vi "Data Producer Worker Template_Read.vi"(0 "Data Producer Worker Template In":refnum<class "Data Producer Worker Template.lvclass">, 7 "Elements to Read (-1: all)":i32=-1) -> (4 "Data Producer Worker Template Out":refnum<class "Data Producer Worker Template.lvclass">)   [LabVIEW 2013, in "Data Producer Worker Template.lvclass"]
uses:
  Data Producer Worker Template.lvclass
  Data Producer Worker Template.lvclass/Data Producer Worker Template.ctl
panel:
  out "Timeout":bool
  out "Elements Remaining":i32
  out "error out":errorcluster
  in  "error in (no error)":errorcluster
  in  "timeout in ms (-1)":i32=-1
  out "Data":dbl[](array[numeric])
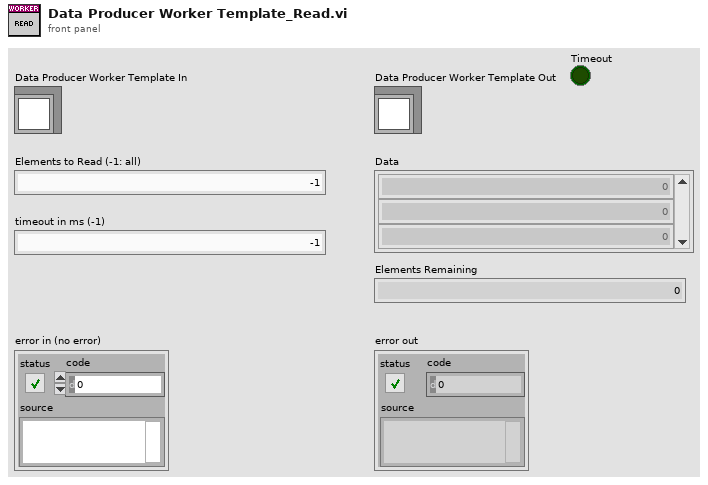
[diagram p1: front panel]
types:
  T1 = typedef "Data Producer Worker Template.lvclass/Data Producer Worker Template_Data Queue.ctl" = refnum<queue>
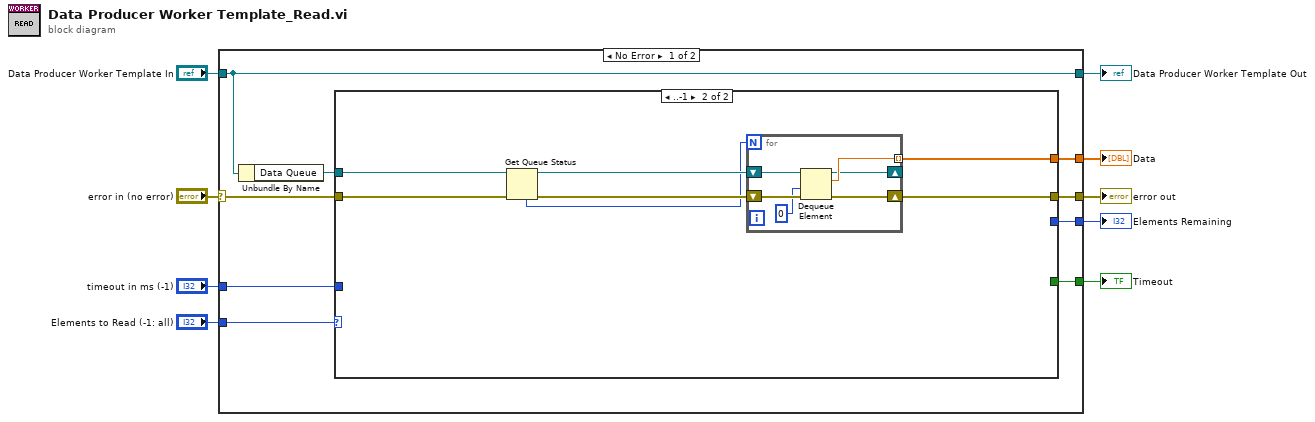
[diagram p0: block diagram]
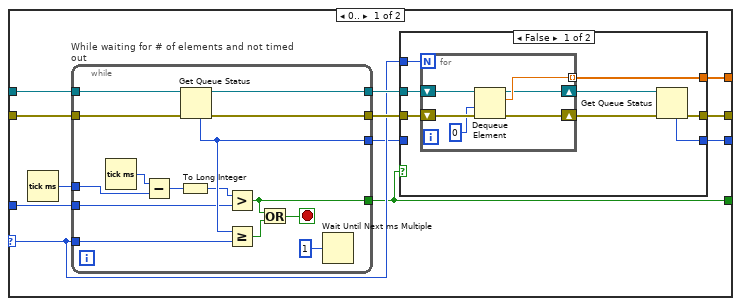
[diagram p2: hidden frame]
diagram:
  n1 = case shown="No Error" "error in (no error)" {
    selector: "error in (no error)" -> [w14 w75]
    tunnel: "Data Producer Worker Template In" -> [w12 w76]
    tunnel: [w17 _] -> w8
    tunnel: "Elements to Read (-1: all)" -> [w16 _]
    tunnel: "timeout in ms (-1)" -> [w15 _]
    tunnel: [w13 w75] -> w4
    tunnel: [w12 w76] -> w3
    tunnel: [w11 _] -> w2
    tunnel: [w10 _] -> w1
    frame No Error {
      n2 = Unbundle By Name(w12) -> ("Data Queue"=w18:T1)
      n3 = case shown="..-1" w16 {
        selector: w16 -> [w23 _]
        tunnel: w18 -> [w26 w65]
        tunnel: [w30 w68] -> w17
        tunnel: w15 -> [w20 _]
        tunnel: w14 -> [w29 w67]
        tunnel: [w28 w63] -> w13
        tunnel: [w24 _] -> w11
        tunnel: [w19 _] -> w10
        frame 0.. {
          n4 = Tick Count (ms)() -> (millisecond timer value=w21:u32)
          n5 = while "While waiting for # of elements and not timed out" {
            tunnel: w29 -> [w45]
            tunnel: [w44] -> w27
            tunnel: w26 -> [w43]
            tunnel: [w42] -> w25
            tunnel: w23 -> [w41]
            tunnel: [w31] -> w19
            tunnel: [w40] -> w22
            tunnel: w21 -> [w36]
            tunnel: w20 -> [w34]
            stop <- w33 stop-if-true
            n6 = Tick Count (ms)() -> (millisecond timer value=w37:u32)
            n7 = Subtract(x=w37, y=w36) -> (x-y=w35:u32)
            n8 = To Long Integer(number=w35) -> (32bit integer=w32:i32)
            n9 = Get Queue Status(queue=w43, error in (no error)=w45) -> (queue out=w42:T1, error out=w44:errorcluster, # elements in queue=w40:i32)  [unwired: 1 in, 5 out]
            n10 = Greater?(x=w32, y=w34) -> (0:w31:bool)
            n11 = Greater Or Equal?(x=w40, y=w41) -> (x >= y?=w39:bool)
            n12 = Or(x=w31, y=w39) -> (x .or. y?=w33:bool)
            n13 = Wait Until Next ms Multiple(millisecond multiple=u32 1) -> ()  [unwired: 1 out]
          }
          n14 = case shown="False" w19 {
            tunnel: [w53 _] -> w30
            tunnel: w23 -> [w52 _]
            tunnel: [w50 w61] -> w28
            tunnel: w27 -> [w48 w61]
            tunnel: w25 -> [w47 _]
            tunnel: [w46 w60] -> w24
            tunnel: w22 -> [_ w60]
            frame False {
              n15 = for {
                N: w52 -> [_]
                tunnel: [w58] -> w53 mode=indexing
                shift-right: [w55] -> w51
                shift-left: w48 -> [w57]
                shift-right: [w56] -> w49
                shift-left: w47 -> [w59]
                n16 = Dequeue Element(queue=w59, timeout in ms (-1)=0, error in (no error)=w57) -> (queue out=w56:T1, element=w58:dbl, error out=w55:errorcluster)  [unwired: 1 out]
              }
              n17 = Get Queue Status(queue=w49, error in (no error)=w51) -> (error out=w50:errorcluster, # elements in queue=w46:i32)  [unwired: 1 in, 6 out]
            }
            frame True {
            }
          }
        }
        frame ..-1 {
          n18 = Get Queue Status(queue=w65, error in (no error)=w67) -> (queue out=w64:T1, error out=w66:errorcluster, # elements in queue=w62:i32)  [unwired: 1 in, 5 out]
          n19 = for {
            N: w62 -> [_]
            tunnel: [w73] -> w68 mode=indexing
            shift-right: [w70] -> w63
            shift-left: w66 -> [w72]
            shift-right: [w71] -> _
            shift-left: w64 -> [w74]
            n20 = Dequeue Element(queue=w74, timeout in ms (-1)=0, error in (no error)=w72) -> (queue out=w71:T1, element=w73:dbl, error out=w70:errorcluster)  [unwired: 1 out]
          }
        }
      }
    }
    frame Error {
    }
  }
  "Data" <- w8
  "error out" <- w4
  "Data Producer Worker Template Out" <- w3
  "Elements Remaining" <- w2
  "Timeout" <- w1
